vi "DSP_read.vi"(1 "inst param":T1) -> (0 "array":dbl[](array[numeric]))   [LabVIEW 2013]
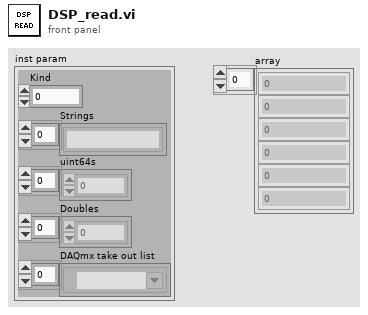
[diagram p1: front panel]
types:
  T1 = cluster{"Kind":u16, "Strings":string[], "uint64s":u64[], "Doubles":dbl[], "DAQmx take out list":refnum<k21>[]}
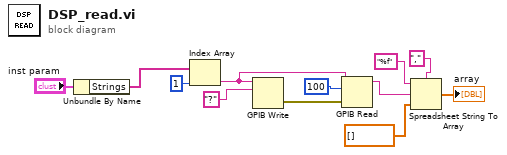
[diagram p0: block diagram]
diagram:
  n1 = Unbundle By Name("inst param") -> ("Strings"=w11:string[])
  n2 = Index Array(array=w11, index=1) -> (element=w8:string)
  n3 = GPIB Write(0:w8, 1:"?") -> (6:w7:errorcluster)  [unwired: 3 in, 1 out]
  n4 = GPIB Read(0:w8, 1:100, 3:w7) -> (5:w5:string)  [unwired: 2 in, 2 out]
  n5 = Spreadsheet String To Array(delimiter (Tab)=",", format string="%f", spreadsheet string=w5, array type (2D Dbl)=dbl[] []) -> (array=→"array":dbl[])
